vi "SUPER PID (F11).vi"(0 "SP Up":bool, 1 "SP Increment":dbl=1.0, 2 "SP Down":bool, 3 "DC Up":bool, 4 "DC Increment":dbl=1.0, 5 "DC Down":bool, 6 "Manual / Auto":bool, 7 "PV":dbl, 8 "P":dbl=1.0 format="%0.2f", 10 "I":dbl=0.1 format="%0.2f", 11 "upper limit":dbl=100.0 format="%0.2f", 12 "D":dbl=0.05 format="%0.2f", 13 "lower limit":dbl format="%0.2f") -> (14 "SP":dbl, 15 "DC":dbl, 16 "CO Bias":dbl, 17 "P out":dbl, 18 "I out":dbl, 19 "D out":dbl)   [LabVIEW 2013]
doc: "This is a SUPER PID which can be used to control a system. The idea of a PID is to control a system by comparing the set point (the system value you want) to the process variable (the current system value), and adjusting the output value (what you output to the system in an attempt to get the process variable to approach the set point. This SUPER PID includes manual/auto selection, bumpless transfer, and anti-reset windup.\n\nThe set point is the value you desire the system to achieve.\n\nThe process variable is the current value of your system, and is usually acquired by an analog input channel of your DAQ device.\n\nP is the Proportional component. This is the amount by which the error gets multiplied. The error is the set point minus the process variable.\n\nI is the Integral component. This is how much the PID output will depend on what has happened in the past.\n\nD is the derivative component. This is how much the PID output will depend on speculation of what will happen in the future.\n\nThe output value is the PID output which is usually generated at an analog output channel of your DAQ device in an attempt to get the process variable equal to the set point.\n\nThe upper limit is the maximum value the PID can output to the system.\n\nThe lower limit is the minimum value the PID can output to the system."
panel:
  # "(Process Variable) Variable"
  # "(Setpoint)"
  # "Note: This function is not designed for control\nloop rates > 1kHz.  The dt calculation has a\nresolution of 1 ms; therefore, loop rates > 1kHz\nwill result in incorrect output for derivative and\nintegral action."
  # "(Duty Cycle; CO, controller output)\n)"
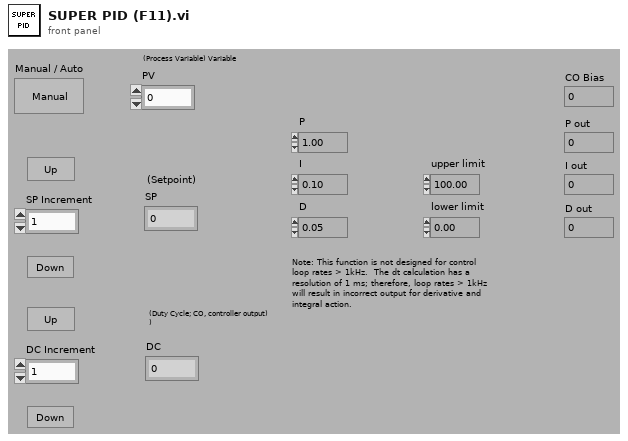
[diagram p1: front panel]
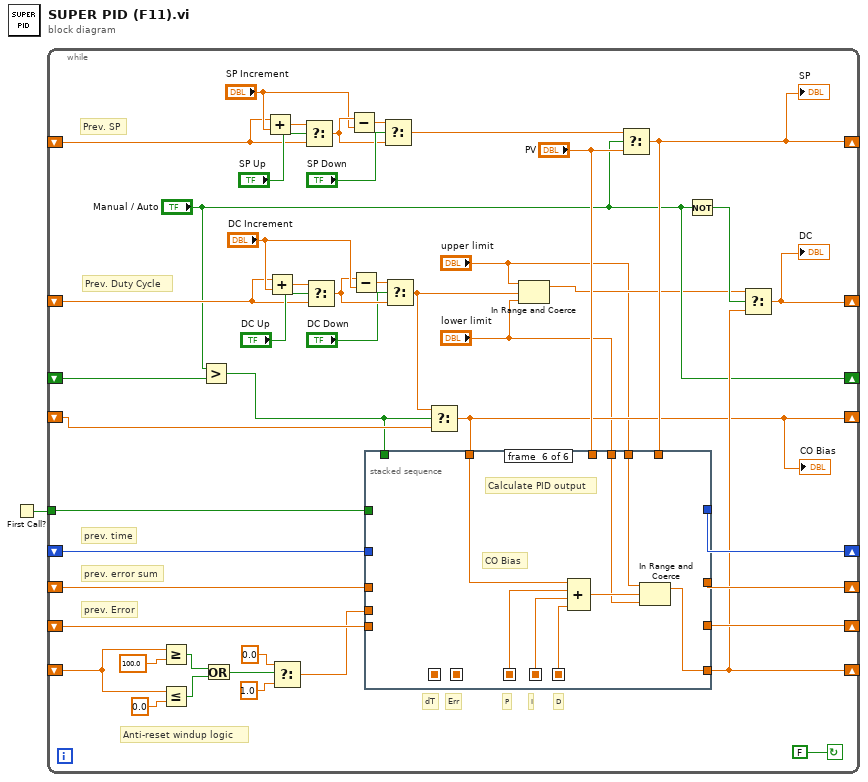
[diagram p0: block diagram]
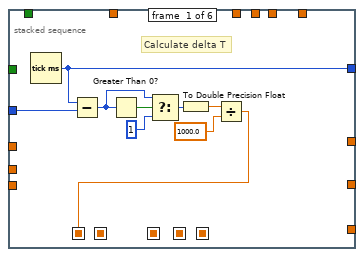
[diagram p2: hidden frame]
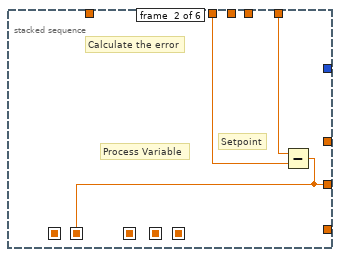
[diagram p3: hidden frame]
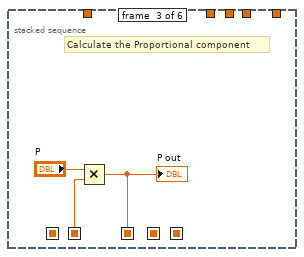
[diagram p4: hidden frame]
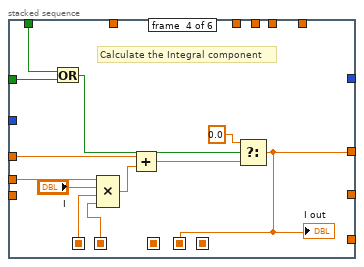
[diagram p5: hidden frame]
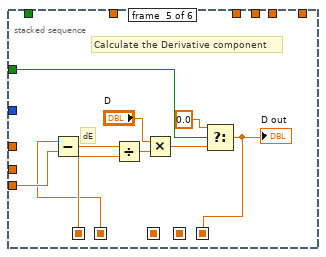
[diagram p6: hidden frame]
diagram:
  n1 = First Call?() -> (First Call?: T/F=w1:bool)
  n2 = while {
    shift-left: _ -> [w42]
    shift-right: [w43] -> _
    shift-left: _ -> [w45]
    shift-right: [w44] -> _
    shift-left: _ -> [w46]
    shift-right: [w47] -> _
    tunnel: w1 -> [w40]
    shift-right: [w15] -> _
    shift-left: _ -> [w24]
    shift-right: [w16] -> _
    shift-left: _ -> [w11]
    shift-right: [w13] -> _
    shift-left: _ -> [w14]
    shift-right: ["Manual / Auto"] -> _
    shift-left: _ -> [w10]
    shift-right: [w6] -> _
    shift-left: _ -> [w8]
    stop <- FALSE continue-if-true
    # "Prev. Duty Cycle"
    # "Prev. SP"
    # "Anti-reset windup logic"
    # "I"
    # "dT"
    # "Err"
    # "D"
    # "P"
    # "prev. error sum"
    # "prev. time"
    # "prev. Error"
    n3 = Greater Or Equal?(x=w14, y=100.0) -> (x >= y?=w37:bool)
    n4 = Less Or Equal?(x=w14, y=0.0) -> (x <= y?=w36:bool)
    n5 = Greater?(x="Manual / Auto", y=w10) -> (0:w7:bool)
    n6 = Or(x=w37, y=w36) -> (x .or. y?=w35:bool)
    n7 = Add(x=w24, y="SP Increment") -> (x+y=w30:dbl)
    n8 = Add(x=w11, y="DC Increment") -> (x+y=w19:dbl)
    n9 = Select(t=0.0, s=w35, f=1.0) -> (s? t:f=w32:dbl)
    n10 = Select(t=w30, s="SP Up", f=w24) -> (s? t:f=w26:dbl)
    n11 = Select(t=w19, s="DC Up", f=w11) -> (s? t:f=w22:dbl)
    n12 = Subtract(x=w26, y="SP Increment") -> (x-y=w31:dbl)
    n13 = Subtract(x=w22, y="DC Increment") -> (x-y=w18:dbl)
    n14 = Select(t=w31, s="SP Down", f=w26) -> (s? t:f=w27:dbl)
    n15 = Select(t=w18, s="DC Down", f=w22) -> (s? t:f=w5:dbl)
    n16 = Select(t=w5, s=w7, f=w8) -> (s? t:f=w6:dbl)
    "CO Bias" <- w6
    n17 = In Range and Coerce(upper limit="upper limit", x=w5, lower limit="lower limit") -> (coerced(x)=w4:dbl)  [unwired: 1 out]
    n18 = Select(t=w27, s="Manual / Auto", f="PV") -> (s? t:f=w15:dbl)
    "SP" <- w15
    n19 = stacked-sequence {
      seq-local: [w48 _ _ _ _ _] -> [_ _ _ w70 w79 _]
      seq-local: [_ w59 _ _ _ _] -> [_ _ w61 w69 w78 _]
      seq-local: [_ _ w60 _ _ _] -> [_ _ _ _ _ w91]
      seq-local: [_ _ _ _ w77 _] -> [_ _ _ _ _ w89]
      seq-local: [_ _ _ w67 _ _] -> [_ _ _ _ _ w90]
      tunnel: [w49 _ _ _ _ _] -> w47
      tunnel: w46 -> [w50 _ _ _ _ _]
      tunnel: w45 -> [_ _ _ w71 _ _]
      tunnel: [_ _ _ w67 _ _] -> w44
      tunnel: [_ w59 _ _ _ _] -> w43
      tunnel: w42 -> [_ _ _ _ w80 _]
      tunnel: [_ _ _ _ _ w88] -> w13
      tunnel: w40 -> [_ _ _ w65 w76 _]
      tunnel: w32 -> [_ _ _ w66 _ _]
      tunnel: w15 -> [_ w58 _ _ _ _]
      tunnel: "PV" -> [_ w57 _ _ _ _]
      tunnel: w6 -> [_ _ _ _ _ w87]
      tunnel: w7 -> [_ _ _ w63 _ _]
      tunnel: "upper limit" -> [_ _ _ _ _ w86]
      tunnel: "lower limit" -> [_ _ _ _ _ w85]
      frame #0 {
        # "Calculate delta T"
        n20 = Tick Count (ms)() -> (millisecond timer value=w49:u32)
        n21 = Subtract(x=w49, y=w50) -> (x-y=w55:u32)
        n22 = Greater Than 0?(x=w55) -> (x > 0?=w56:bool)
        n23 = Select(t=w55, s=w56, f=u32 1) -> (s? t:f=w52:u32)
        n24 = To Double Precision Float(number=w52) -> (double precision float=w51:dbl)
        n25 = Divide(x=w51, y=1000.0) -> (x/y=w48:dbl)
      }
      frame #1 {
        # "Process Variable"
        # "Setpoint"
        # "Calculate the error"
        n26 = Subtract(x=w58, y=w57) -> (x-y=w59:dbl)
      }
      frame #2 {
        # "Calculate the Proportional component"
        n27 = Multiply(x="P", y=w61) -> (x*y=w60:dbl)
        "P out" <- w60
      }
      frame #3 {
        # "Calculate the Integral component"
        n28 = Or(x=w63, y=w65) -> (x .or. y?=w64:bool)
        n29 = Compound Arithmetic op=MULTIPLY(w66, "I", w70, w69) -> (w74:dbl)
        n30 = Add(x=w71, y=w74) -> (x+y=w72:dbl)
        n31 = Select(t=0.0, s=w64, f=w72) -> (s? t:f=w67:dbl)
        "I out" <- w67
      }
      frame #4 {
        # "dE"
        # "Calculate the Derivative component"
        n32 = Subtract(x=w78, y=w80) -> (x-y=w81:dbl)
        n33 = Divide(x=w81, y=w79) -> (x/y=w82:dbl)
        n34 = Multiply(x="D", y=w82) -> (x*y=w84:dbl)
        n35 = Select(t=0.0, s=w76, f=w84) -> (s? t:f=w77:dbl)
        "D out" <- w77
      }
      frame #5 {
        # "CO Bias"
        # "Calculate PID output"
        n36 = Compound Arithmetic op=ADD(w87, w91, w90, w89) -> (w92:dbl)
        n37 = In Range and Coerce(upper limit=w86, x=w92, lower limit=w85) -> (coerced(x)=w88:dbl)  [unwired: 1 out]
      }
    }
    n38 = Not(x="Manual / Auto") -> (.not. x?=w17:bool)
    n39 = Select(t=w4, s=w17, f=w13) -> (s? t:f=w16:dbl)
    "DC" <- w16
  }
